vi "moveStageABS.vi"(1 "absolute pos (mm)":dbl, 2 "axisIdx":i32, 3 "System no.":i32=1 min=1 max=4 step=1) -> (0 "Stopped":bool)   [LabVIEW 2015]
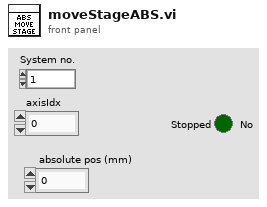
[diagram p1: front panel]
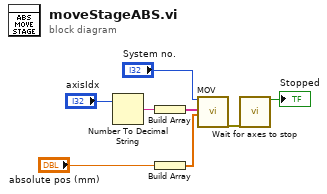
[diagram p0: block diagram]
diagram:
  n1 = Number To Decimal String(number="axisIdx") -> (decimal integer string=w6:string)  [unwired: 1 in]
  n2 = Build Array(w6) -> (w3:string[])
  n3 = Build Array("absolute pos (mm)") -> (w2:dbl[])
  n4 = call "MOV.vi"("System no."="System no.", "Axes to move"=w3, "Position values"=w2) -> ("error out"=w5:errorcluster)  [unwired: 16 in]
  n5 = call "Wait for axes to stop.vi"("error in"=w5) -> ("Stopped"=→"Stopped":bool)  [unwired: 6 in, 12 out]
